vi "RFSG Test Signal Calibration.vi"() -> ()   [LabVIEW 2017]
doc: "Demonstrates how to generate a frequency sweep at a specified power level."
uses:
  <vilib>/Utility/error.llb/DialogType.ctl
  <vilib>/Analysis/1siggen.llb/Ramp Pattern by Delta.vi
  <instrlib>/ni568x/ni568x.llb/ni568x Initialize - IVI.vi
  <instrlib>/ni568x/ni568x.llb/ni568x Read.vi
  Instance           4 28Saved   RFSG Frequency Sweep .vi
  <vilib>/Analysis/NI_AALBase.lvlib
  <vilib>/Utility/file.llb/Write Delimited Spreadsheet (DBL).vi
panel:
  out "Array":dbl[](array[numeric])
  in  "Resource Name 2":refnum<k15>
  in  "Units":i32(ring)=1 caption="measurement units (dBm)" items=["dBm"=1, "Watts"=4, "mWatts"=1001, "uWatts"=1002]
  out "Reading":dbl
  in  "Dwell in Each Step (s)":dbl=1.0 format="%#.6p"
  in  "Delta":dbl=50000000.0 format="%#_6p"
  in  "End Frequency (Hz)":dbl=1010000000.0 format="%#.3p"
  in  "Start Frequency (Hz)":dbl=990000000.0 format="%#.3p"
  in  "Power Level (dBm)":dbl=-5.0 format="%.2f"
  in  "Resource Name":refnum<k15>="RFSG"
  in  "Stop":bool
  out "Current Frequency (Hz)":dbl format="%#_7p"
  # "Frequency Sweep Parameters"
  # "In order to configure new settings you must stop the VI using \nthe Stop button and then run the example with the new settings."
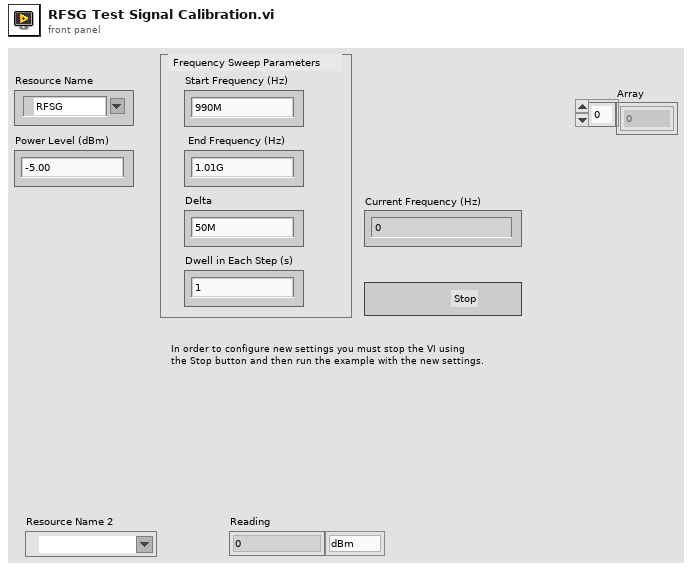
[diagram p1: front panel]
types:
  T1 = typedef "DialogType.ctl" = u16
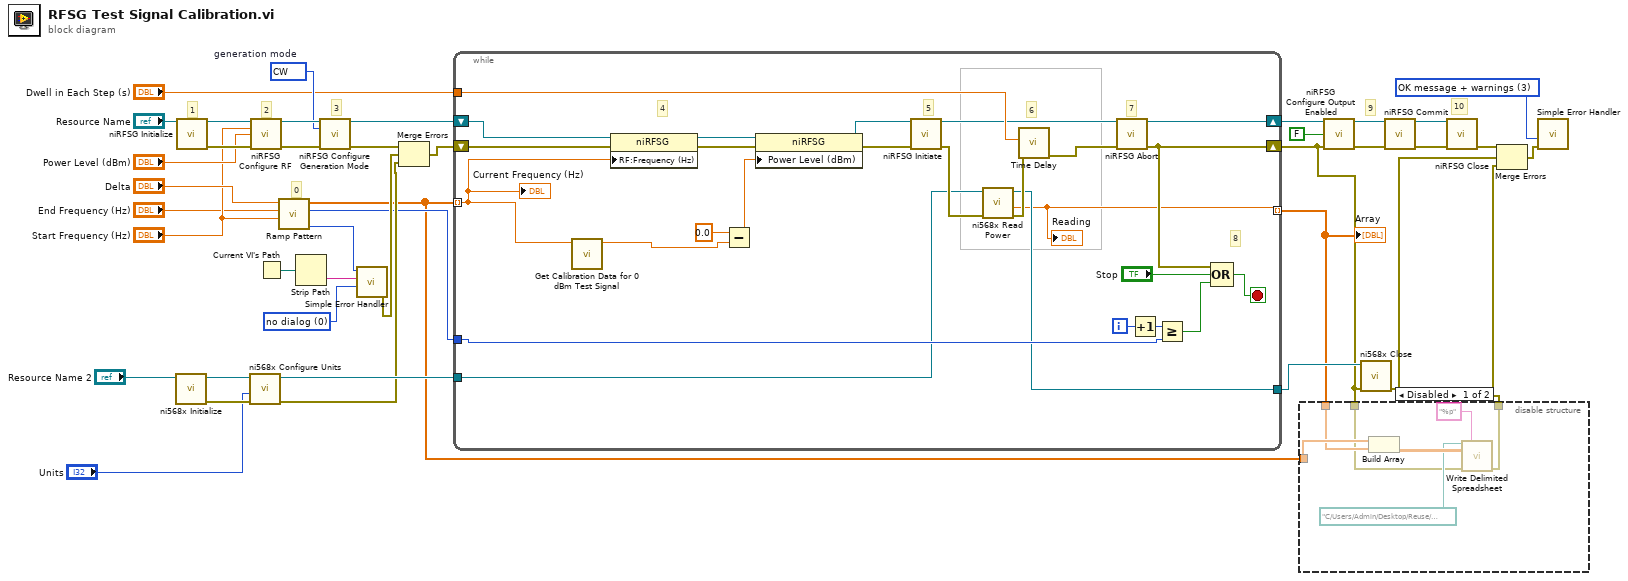
[diagram p0: block diagram]
diagram:
  w16 = T1 3 items=["no dialog", "OK message", "continue or stop message", "OK message + warnings", "continue/stop + warnings"] ("type of dialog (OK msg:1)")
  w22 = 1000 items=["CW"=1000, "Arb Waveform"=1001, "Script"=1002]  # generation mode
  w38 = T1 0 items=["no dialog", "OK message", "continue or stop message", "OK message + warnings", "continue/stop + warnings"] ("type of dialog (OK msg:1)")
  # "9"
  # "3"
  # "0"
  # "10"
  # "2"
  # "1"
  n1 = call-poly <instrlib>:"ni568x Initialize.vi"("resource name"="Resource Name 2") -> ("error out"=w14:errorcluster, "instrument handle"=w15:refnum<k15>)  [unwired: 9 in]
  n2 = call <instrlib>:"niRFSG Initialize.vi"("resource name"="Resource Name") -> ("instrument handle"=w36:refnum<k15>, "error out"=w37:errorcluster)  [unwired: 13 in]
  n3 = call <instrlib>:"ni568x Configure Units.vi"("error in"=w14, "units"="Units", "instrument handle"=w15) -> ("error out"=w10:errorcluster, "instrument handle out"=w11:refnum<k15>)  [unwired: 7 in]
  n4 = call <instrlib>:"niRFSG Configure RF.vi"("instrument handle"=w36, "frequency (Hz)"="Start Frequency (Hz)", "power level (dBm)"="Power Level (dBm)", "error in"=w37) -> ("instrument handle out"=w26:refnum<k15>, "error out"=w24:errorcluster)  [unwired: 10 in]
  n5 = Current VI's Path() -> (path=w41:path)
  n6 = call-poly <vilib>:"Ramp Pattern.vi"("start"="Start Frequency (Hz)", "end"="End Frequency (Hz)", "delta"="Delta") -> ("error"=w39:i32, "samples"=w5:i32, "Ramp Pattern"=w4:dbl[])  [unwired: 6 in]
  n7 = Strip Path(path=w41) -> (name=w40:string)  [unwired: 1 out]
  n8 = call <instrlib>:"niRFSG Configure Generation Mode.vi"("instrument handle"=w26, "generation mode"=w22, "error in"=w24) -> ("instrument handle out"=w25:refnum<k15>, "error out"=w23:errorcluster)  [unwired: 11 in]
  n9 = call <vilib>:"Simple Error Handler.vi"("error code (no error:0)"=w39, "error source (\" \")"=w40, "type of dialog (OK msg:1)"=w38) -> ("error out"=w35:errorcluster)  [unwired: 2 in, 4 out]
  n10 = Merge Errors(w23, w35, w10) -> (w34:errorcluster)
  n11 = while {
    shift-right: [w54] -> w1
    shift-left: w34 -> [w65]
    tunnel: "Dwell in Each Step (s)" -> [w62]
    shift-right: [w56] -> w32
    shift-left: w25 -> [w63]
    tunnel: w4 -> [w48] mode=indexing
    tunnel: w5 -> [w61]
    tunnel: w11 -> [w51]
    tunnel: [w50] -> w9
    tunnel: [w49] -> w3 mode=indexing
    i -> [w60]
    stop <- w67 stop-if-true
    # "7"
    # "4"
    # "8"
    # "6"
    # "5"
    n12 = call "Get Calibration Data for 0 dBm Test Signal.vi"("Carrier Frequency"=w48) -> ("Calibration Data"=w47:dbl)  [unwired: 9 in, 1 out]
    n13 = property class="niRFSG"(reference=w63, error in=w65, "RF:Frequency (Hz)"=w48) -> (reference out=w45:refnum<k15>, error out=w58:errorcluster)
    n14 = Subtract(x=0.0, y=w47) -> (x-y=w43:dbl)
    n15 = property class="niRFSG"(reference=w45, error in=w58, "Power Level (dBm)"=w43) -> (reference out=w44:refnum<k15>, error out=w46:errorcluster)
    n16 = call <instrlib>:"niRFSG Initiate.vi"("instrument handle"=w44, "error in"=w46) -> ("instrument handle out"=w57:refnum<k15>, "error out"=w53:errorcluster)  [unwired: 12 in]
    n17 = call-poly <instrlib>:"ni568x Read Power.vi"("error in"=w53, "instrument handle"=w51) -> ("error out"=w52:errorcluster, "power"=w49:dbl, "instrument handle out"=w50:refnum<k15>)  [unwired: 7 in]
    "Reading" <- w49
    n18 = call "Time Delay"("error in (no error)"=w52, "Delay Time (s)"=w62) -> ("error out"=w55:errorcluster)  [unwired: 9 in]
    n19 = call <instrlib>:"niRFSG Abort.vi"("instrument handle"=w57, "error in"=w55) -> ("instrument handle out"=w56:refnum<k15>, "error out"=w54:errorcluster)  [unwired: 12 in]
    n20 = Increment(x=w60) -> (x+1=w59:i32)
    n21 = Greater Or Equal?(x=w59, y=w61) -> (x >= y?=w66:bool)
    n22 = Compound Arithmetic op=OR(w54, "Stop", w66) -> (w67:bool)
    "Current Frequency (Hz)" <- w48
  }
  "Array" <- w3
  n23 = disable-structure shown="Disabled" {
    disable-tunnel: w4 -> [w74 _]
    disable-tunnel: w3 -> [w73 _]
    disable-tunnel: [w69 _] -> w2
    disable-tunnel: w1 -> [w68 _]
    frame Disabled {
      n24 = Build Array(w74, w73) -> (w72:dbl[][])
      n25 = call-poly <vilib>:"Write Delimited Spreadsheet.vi"("file path (dialog if empty)"=path "C:/Users/Admin/Desktop/Reuse/Scanning Speed PXIe 5668/Calibration Data.txt", "format (%.3f)"="%p", "2D data"=w72, "error in (no error)"=w68) -> ("error out"=w69:errorcluster)  [unwired: 10 in, 1 out]
    }
    frame Enabled {
    }
  }
  n26 = call <instrlib>:"niRFSG Configure Output Enabled.vi"("instrument handle"=w32, "output enabled"=FALSE ("output enable"), "error in"=w1) -> ("instrument handle out"=w31:refnum<k15>, "error out"=w30:errorcluster)  [unwired: 11 in]
  n27 = call <instrlib>:"ni568x Close.vi"("error in"=w1, "instrument handle"=w9) -> ("error out"=w6:errorcluster)  [unwired: 9 in]
  n28 = call <instrlib>:"niRFSG Commit.vi"("instrument handle"=w31, "error in"=w30) -> ("instrument handle out"=w29:refnum<k15>, "error out"=w28:errorcluster)  [unwired: 12 in]
  n29 = call <instrlib>:"niRFSG Close.vi"("instrument handle"=w29, "error in"=w28) -> ("error out"=w8:errorcluster)  [unwired: 13 in]
  n30 = Merge Errors(w8, w6, w2) -> (w7:errorcluster)
  n31 = call <vilib>:"Simple Error Handler.vi"("type of dialog (OK msg:1)"=w16, "error in (no error)"=w7) -> ()  [unwired: 3 in, 5 out]
